vi "Run Test.vi"(8 "error in (no error)":errorcluster, 11 "Test Template in":refnum<class "DPM Failure Test.lvclass">) -> (0 "error out":errorcluster, 1 "Fail Codes":string[](array[string]), 2 "Tests Passed":bool[](array[boolean]), 3 "Test Template out":refnum<class "DPM Failure Test.lvclass">)   [LabVIEW 2015, in "DPM Failure Test.lvclass"]
uses:
  DPM Failure Test.lvclass
  Examples/DPM Failure Test/Application/Application/Class/typedefs/Instrument Selector -- Enum.ctl
  Classes/Instruments/AC Power Supply/AC Power Supply/Class/AC Power Supply.lvclass
  Classes/Instruments/Digital Power Meter/Digital Power Meter/Class/Digital Power Meter.lvclass
  Test Class/Test Class.lvclass
  Classes/Application/Class/Application.lvclass
  Examples/DPM Failure Test/Application/Application/Class/DPM Failure Test.lvclass
  <vilib>/Cree, Inc/Cree Test Framework/Core Launcher/Core Launcher.lvlib
  <vilib>/Cree, Inc/Cree Test Framework/Classes/Data/Data Repo/Class/Data Repo.lvclass
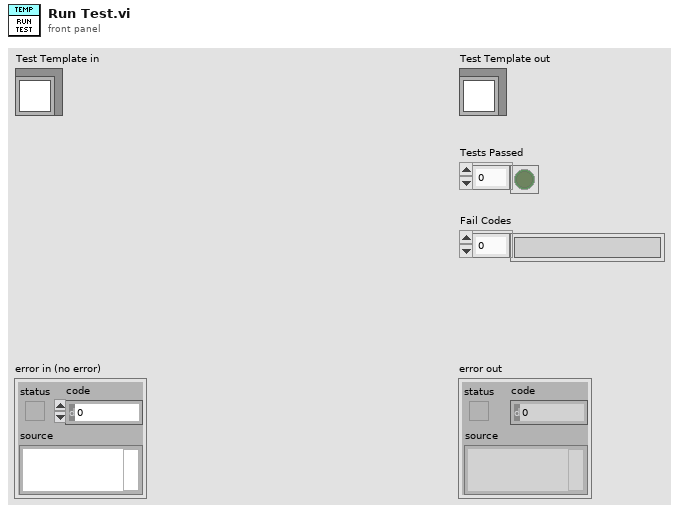
[diagram p1: front panel]
types:
  T1 = typedef "DPM Failure Test.lvlib/DPM Failure Test.lvclass/Instrument Selector -- Enum.ctl" = enum16{"AC Power Supply", "DPM"}
  T2 = typedef "Application.lvlib/App Properties.lvclass/Class Properties -- Cluster.ctl" = cluster{"UUT Info":T3[], "Test Information":refnum<vi>, "Test Complete Event":refnum<user-event>, "Shop Floor System":refnum<class "Shop Floor System.lvclass">, "Gold Board":refnum<class "Golden Board.lvclass">, "Test Recipe":refnum<class "Test Recipe.lvclass">, "Instruments":refnum<class "Instrument.lvclass">[], "Mode":T4, "Test Results":cluster{"Pass":bool[], "Fail Codes":string[]}, "Station Config":refnum<class "Station Config.lvclass">}
  T3 = typedef "Application.lvlib/App Properties.lvclass/UUT Reference -- Cluster.ctl" = cluster{"Serial Number Reference":refnum<vi>, "Status Message Reference":refnum<vi>}
  T4 = typedef "Application.lvlib/Application.lvclass/Op Mode -- Enum.ctl" = u16
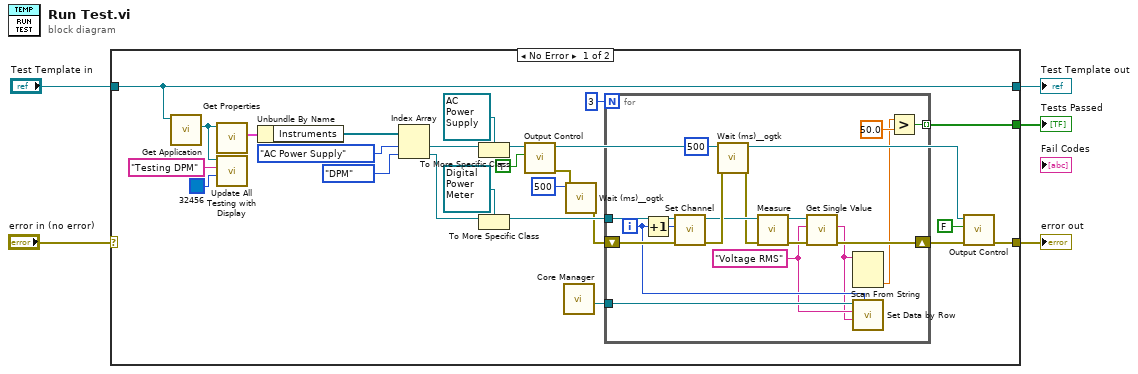
[diagram p0: block diagram]
diagram:
  n1 = case shown="No Error" "error in (no error)" {
    selector: "error in (no error)" -> [_ w48]
    tunnel: [w8 w48] -> w2
    tunnel: "Test Template in" -> [w29 w47]
    tunnel: [w29 w47] -> w3
    tunnel: [w11 _] -> w1
    frame No Error {
      n2 = call "Get Application.vi"("Test Class in"=w29) -> ("Application.lvlib:Application.lvclass"=w26:refnum<class "Application.lvclass">)  [unwired: 9 in, 1 out]
      n3 = call "Get Properties.vi"("Acrobat Template in"=w26) -> ("Class Properties"=w25:T2)  [unwired: 8 in, 2 out]
      n4 = call "Update All Testing with Display.vi"("BG Color"=u32 32456, "Message ('')"="Testing DPM", "Application in"=w26) -> ()  [unwired: 7 in, 2 out]
      n5 = Unbundle By Name(w25) -> ("Instruments"=w24:refnum<class "Instrument.lvclass">[])
      n6 = Index Array(array=w24, index #1=Instrument_Selector_--_Enum."AC Power Supply" ("Instrument"), index #2=Instrument_Selector_--_Enum."DPM" ("Instrument")) -> (element #1=w21:refnum<class "Instrument.lvclass">, element #2=w19:refnum<class "Instrument.lvclass">)
      n7 = To More Specific Class(target class=refnum<class "AC Power Supply.lvclass"> refnum ("AC Power Supply.lvlib:AC Power Supply.lvclass"), reference=w21) -> (specific class reference=w6:refnum<class "AC Power Supply.lvclass">)  [unwired: 1 in, 1 out]
      n8 = To More Specific Class(target class=refnum<class "Digital Power Meter.lvclass"> refnum ("Digital Power Meter.lvlib:Digital Power Meter.lvclass"), reference=w19) -> (specific class reference=w14:refnum<class "Digital Power Meter.lvclass">)  [unwired: 1 in, 1 out]
      n9 = call-dynamic "Output Control.vi"("Enabled"=TRUE, "Acrobat Template in"=w6) -> ("error out"=w16:errorcluster)  [unwired: 8 in, 1 out]
      n10 = call <vilib>:"Core Manager.vi"() -> ("Data Repo"=w10:refnum<class "Data Repo.lvclass">)  [unwired: 8 in, 3 out]
      n11 = call <userlib>:"Wait (ms)__ogtk.vi"("error in (no error)"=w16, "milliseconds to wait"=u32 500) -> ("error out"=w13:errorcluster)  [unwired: 8 in, 1 out]
      n12 = for {
        N: 3 -> [_]
        shift-right: [w38] -> w9
        shift-left: w13 -> [w37]
        tunnel: [w34] -> w11 mode=indexing
        tunnel: w10 -> [w33]
        tunnel: w14 -> [w46]
        i -> [w32]
        w31 = "Voltage RMS" ("Filter")
        n13 = Increment(x=w32) -> (x+1=w45:i32)
        n14 = call-dynamic "Set Channel.vi"("error in (no error)"=w37, "Channel"=w45, "Acrobat Template in"=w46) -> ("error out"=w43:errorcluster, "Acrobat Template out"=w42:refnum<class "Digital Power Meter.lvclass">)  [unwired: 7 in]
        n15 = call <userlib>:"Wait (ms)__ogtk.vi"("error in (no error)"=w43, "milliseconds to wait"=u32 500) -> ("error out"=w41:errorcluster)  [unwired: 8 in, 1 out]
        n16 = call-dynamic "Measure.vi"("error in (no error)"=w41, "Acrobat Template in"=w42) -> ("error out"=w39:errorcluster, "Acrobat Template out"=w40:refnum<class "Digital Power Meter.lvclass">)  [unwired: 8 in]
        n17 = call "Get Single Value.vi"("error in (no error)"=w39, "Filter"=w31, "Acrobat Template in"=w40) -> ("error out"=w38:errorcluster, "Data"=w30:string)  [unwired: 6 in, 1 out]
        n18 = Scan From String(input string=w30) -> (output 1=w35:dbl)  [unwired: 4 in, 3 out]
        n19 = call <vilib>:"Set Data by Row.vi"("Row"=w32, "Value"=w30, "Header"=w31, "Acrobat Template in"=w33) -> ()  [unwired: 6 in, 2 out]
        n20 = Greater?(x=w35, y=50.0) -> (0:w34:bool)
      }
      n21 = call-dynamic "Output Control.vi"("error in (no error)"=w9, "Enabled"=FALSE, "Acrobat Template in"=w6) -> ("error out"=w8:errorcluster)  [unwired: 7 in, 1 out]
    }
    frame Error {
    }
  }
  "error out" <- w2
  "Test Template out" <- w3
  "Tests Passed" <- w1
